vi "BinaryMono_SliderControl.vi"(7 "NewVal":T1, 8 "Error In":errorcluster, 9 "Look For":T2(ring), 10 "Threshold Range Gray":cluster{dbl, dbl}, 11 "Cluster in":refnum<vi>) -> (0 "Error Out":errorcluster, 3 "BinaryMonoParam Out":T1)   [LabVIEW 2019]
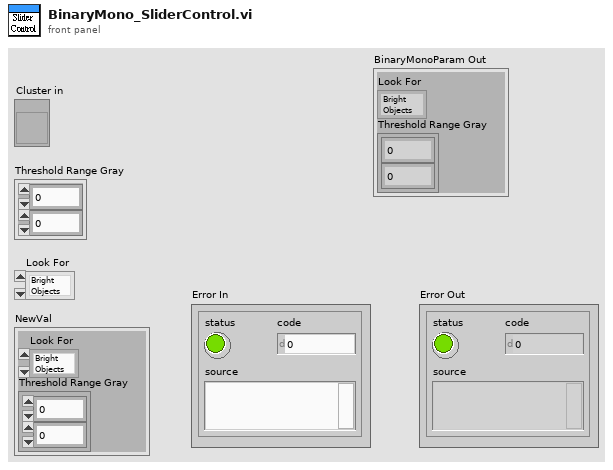
[diagram p1: front panel]
types:
  T1 = cluster{"Look For":enum16{"Bright Objects", "Dark Objects", "Gray Objects"}, "Threshold Range Gray":cluster{dbl, dbl}}
  T2 = enum16{"Bright Objects", "Dark Objects", "Gray Objects"}
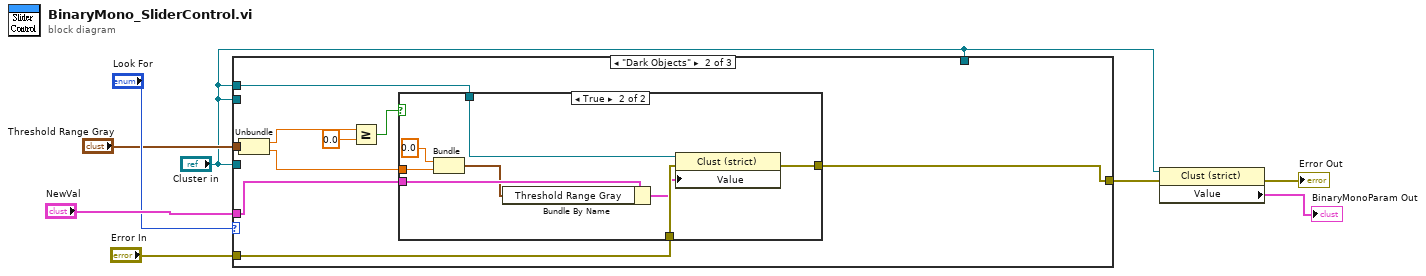
[diagram p0: block diagram]
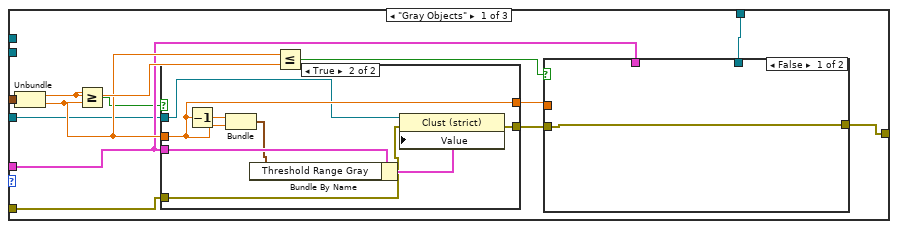
[diagram p2: hidden frame]
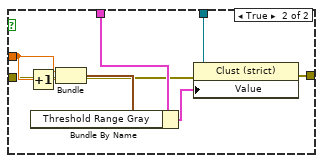
[diagram p3: hidden frame]
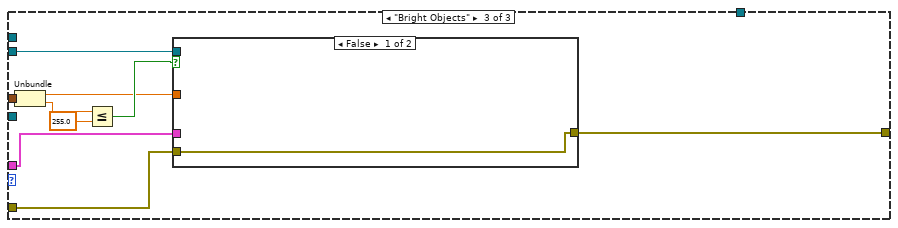
[diagram p6: hidden frame]
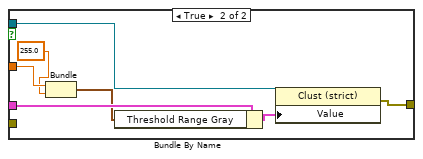
[diagram p7: hidden frame]
diagram:
  n1 = case shown="\"Dark Objects\"" "Look For" {
    tunnel: "Threshold Range Gray" -> [w18 w48 w66]
    tunnel: "NewVal" -> [w15 w45 w65]
    tunnel: "Cluster in" -> [w13 _ _]
    tunnel: "Cluster in" -> [w12 _ _]
    tunnel: "Cluster in" -> [_ w42 _]
    tunnel: "Cluster in" -> [_ _ w60]
    tunnel: [w9 w40 w59] -> w4
    tunnel: "Error In" -> [w11 w41 w58]
    frame "Gray Objects" {
      n2 = Unbundle(w18) -> (w17:dbl, w16:dbl)
      n3 = Greater Or Equal?(x=w17, y=w16) -> (x >= y?=w14:bool)
      n4 = case shown="True" w14 {
        tunnel: w16 -> [w31 w38]
        tunnel: [w31 w38] -> w19
        tunnel: w15 -> [_ w37]
        tunnel: w13 -> [_ w34]
        tunnel: w11 -> [w30 w33]
        tunnel: [w30 w32] -> w10
        frame False {
        }
        frame True {
          n5 = Decrement(x=w38) -> (x-1=w39:dbl)
          n6 = Bundle(w39, w38) -> (w36:cluster{dbl, dbl})  [unwired: 1 in]
          n7 = Bundle By Name(cluster=w37, "Threshold Range Gray"=w36) -> (w35:T1)
          n8 = property class="Clust (strict)"(reference=w34, error in=w33, "Value"=w35) -> (error out=w32:errorcluster)  [unwired: 1 out]
        }
      }
      n9 = Less Or Equal?(x=w16, y=w17) -> (x <= y?=w20:bool)
      n10 = case shown="False" w20 {
        tunnel: w19 -> [_ w29]
        tunnel: w15 -> [_ w26]
        tunnel: w12 -> [_ w24]
        tunnel: w10 -> [w21 w23]
        tunnel: [w21 w22] -> w9
        frame False {
        }
        frame True {
          n11 = Increment(x=w29) -> (x+1=w28:dbl)
          n12 = Bundle(w29, w28) -> (w27:cluster{dbl, dbl})  [unwired: 1 in]
          n13 = Bundle By Name(cluster=w26, "Threshold Range Gray"=w27) -> (w25:T1)
          n14 = property class="Clust (strict)"(reference=w24, error in=w23, "Value"=w25) -> (error out=w22:errorcluster)  [unwired: 1 out]
        }
      }
    }
    frame "Dark Objects" {
      n15 = Unbundle(w48) -> (w47:dbl, w43:dbl)
      n16 = Greater Or Equal?(x=w47, y=0.0) -> (x >= y?=w44:bool)
      n17 = case shown="True" w44 {
        tunnel: w45 -> [_ w57]
        tunnel: w43 -> [_ w55]
        tunnel: w42 -> [_ w53]
        tunnel: w41 -> [w49 w52]
        tunnel: [w49 w51] -> w40
        frame False {
        }
        frame True {
          n18 = Bundle("y"=0.0, w55) -> (w54:cluster{"y":dbl, dbl})  [unwired: 1 in]
          n19 = Bundle By Name(cluster=w57, "Threshold Range Gray"=w54) -> (w50:T1)
          n20 = property class="Clust (strict)"(reference=w53, error in=w52, "Value"=w50) -> (error out=w51:errorcluster)  [unwired: 1 out]
        }
      }
    }
    frame "Bright Objects" {
      n21 = Unbundle(w66) -> (w61:dbl, w64:dbl)
      n22 = Less Or Equal?(x=w64, y=255.0) -> (x <= y?=w62:bool)
      n23 = case shown="False" w62 {
        tunnel: w65 -> [_ w74]
        tunnel: w61 -> [_ w72]
        tunnel: w60 -> [_ w69]
        tunnel: [w67 w68] -> w59
        tunnel: w58 -> [w67 _]
        frame False {
        }
        frame True {
          n24 = Bundle(w72, "y"=255.0) -> (w73:cluster{dbl, "y":dbl})  [unwired: 1 in]
          n25 = Bundle By Name(cluster=w74, "Threshold Range Gray"=w73) -> (w70:T1)
          n26 = property class="Clust (strict)"(reference=w69, "Value"=w70) -> (error out=w68:errorcluster)  [unwired: 1 in, 1 out]
        }
      }
    }
  }
  n27 = property class="Clust (strict)"(reference="Cluster in", error in=w4) -> (error out=→"Error Out":errorcluster, "Value"=→"BinaryMonoParam Out":T1)  [unwired: 1 out]
